vi "View Direction Write.vi"(6 "Control Ref Queue":T1, 8 "error in (no error)":errorcluster, 9 "View Direction":T2(ring), 11 "3D Plot.lvclass in":refnum<class "3D Plot.lvclass">) -> (0 "error out":errorcluster, 3 "3D Plot.lvclass out":refnum<class "3D Plot.lvclass">)   [LabVIEW 2020, in "3D Plot.lvclass"]
uses:
  3D Plot.lvclass
  3DMathPlot Ctrl Act Queue.ctl
  3DMathPlot Ctrl Act Cluster.ctl
  3DMathPlot State Class.ctl
  3D Plot.lvclass/3D Plot.ctl
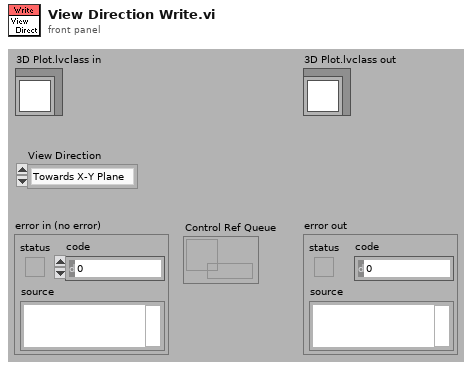
[diagram p1: front panel]
types:
  T1 = typedef "3DMathPlot Ctrl Act Queue.ctl" = refnum<queue>
  T2 = enum32{"Towards X-Y Plane", "Towards X-Z Plane", "Towards Y-Z Plane", "User Defined"}
  T3 = typedef "3DMathPlot Ctrl Act Cluster.ctl" = cluster{"3D Picture Control":refnum<vi>, "Render Window Refnum":refnum<vi>, "XY Graph":refnum<vi>, "Intensity Graph":refnum<vi>, "Color Legend Palette":refnum<vi>, "Projection Palette":refnum<vi>, "XControl  Ref":refnum<vi>, "Facade Ref":refnum<vi>, "Export Image Ref":refnum<vi>, "Clear Data Flag":bool, "Display State Change Class":T4}
  T4 = typedef "3DMathPlot State Class.ctl" = enum16{"Update All Objects (Undo)", "Update Light Object Only", "Update Axis Object Only", "Update Plot Object Only", "Update Cursor Object Only", "Update Axis Plot Cursor Objects", "No Update"}
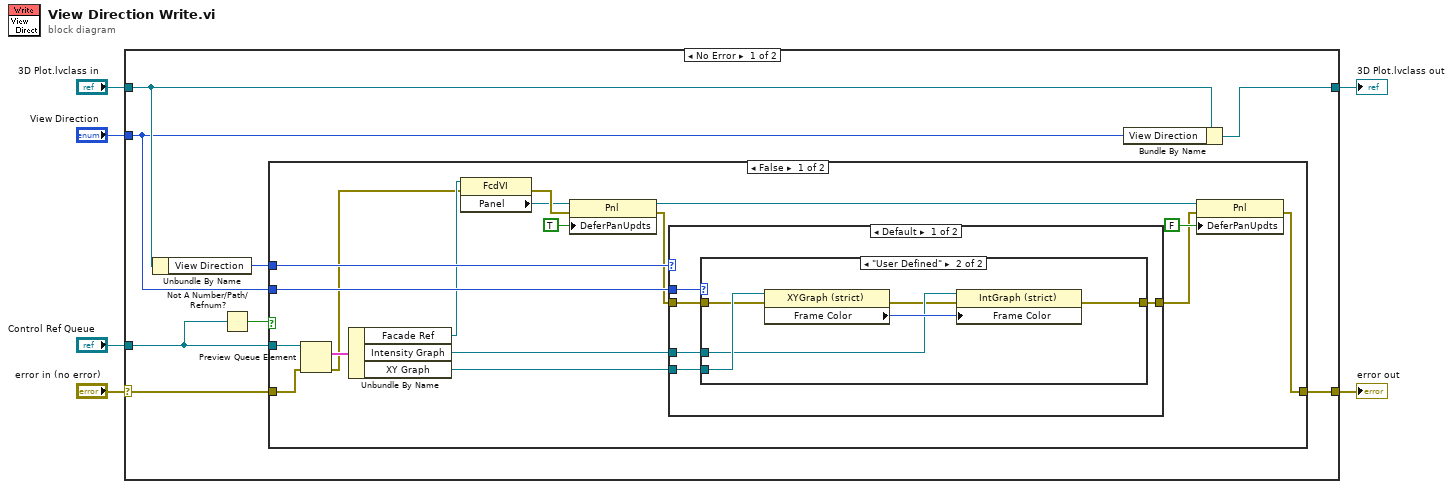
[diagram p0: block diagram]
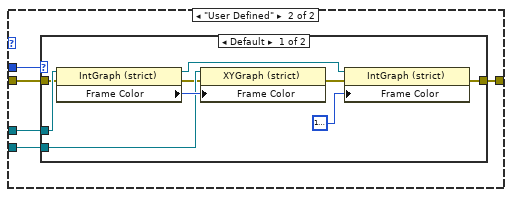
[diagram p3: hidden frame]
diagram:
  n1 = case shown="No Error" "error in (no error)" {
    selector: "error in (no error)" -> [w11 w60]
    tunnel: "View Direction" -> [w9 _]
    tunnel: "3D Plot.lvclass in" -> [w13 w61]
    tunnel: [w14 w61] -> w4
    tunnel: [w7 w60] -> w2
    tunnel: "Control Ref Queue" -> [w8 _]
    frame No Error {
      n2 = Unbundle By Name(w13) -> ("View Direction"=w10:T2)
      n3 = Not A Number/Path/Refnum?(number/path/refnum=w8) -> (NaN/Path/Refnum?=w12:bool)
      n4 = case shown="False" w12 {
        tunnel: w8 -> [w30 _]
        tunnel: w11 -> [w29 w59]
        tunnel: w10 -> [w28 _]
        tunnel: w9 -> [w27 _]
        tunnel: [w15 w59] -> w7
        frame False {
          n5 = Preview Queue Element(queue=w30, error in (no error)=w29) -> (element=w31:T3, error out=w18:errorcluster)  [unwired: 3 out]
          n6 = Unbundle By Name(w31) -> ("Facade Ref"=w23:refnum<vi>, "Intensity Graph"=w20:refnum<vi>, "XY Graph"=w19:refnum<vi>)
          n7 = property class="FcdVI"(reference=w23, error in=w18) -> (error out=w26:errorcluster, "Panel"=w24:refnum<vi>)  [unwired: 1 out]
          n8 = property class="Pnl"(reference=w24, error in=w26, "DeferPanUpdts"=TRUE ("Defer Panel Updates")) -> (reference out=w21:refnum<vi>, error out=w17:errorcluster)
          n9 = case shown="Default" w28 {
            tunnel: w27 -> [w36 w48]
            tunnel: w20 -> [w34 w47]
            tunnel: w19 -> [w35 w46]
            tunnel: w17 -> [w33 w45]
            tunnel: [w32 w44] -> w16
            frame Default {
              n10 = case shown="\"User Defined\"" w36 {
                tunnel: w35 -> [_ w42]
                tunnel: w34 -> [_ w41]
                tunnel: w33 -> [w37 w40]
                tunnel: [w37 w38] -> w32
                frame Default {
                }
                frame "User Defined" {
                  n11 = property class="XYGraph (strict)"(reference=w42, error in=w40) -> (error out=w39:errorcluster, "Frame Color"=w43:u32)  [unwired: 1 out]
                  n12 = property class="IntGraph (strict)"(reference=w41, error in=w39, "Frame Color"=w43) -> (error out=w38:errorcluster)  [unwired: 1 out]
                }
              }
            }
            frame "User Defined" {
              n13 = case shown="Default" w48 {
                tunnel: w47 -> [w57 _]
                tunnel: w46 -> [w55 _]
                tunnel: w45 -> [w54 w58]
                tunnel: [w49 w58] -> w44
                frame Default {
                  n14 = property class="IntGraph (strict)"(reference=w57, error in=w54) -> (reference out=w51:refnum<vi>, error out=w53:errorcluster, "Frame Color"=w56:u32)
                  n15 = property class="XYGraph (strict)"(reference=w55, error in=w53, "Frame Color"=w56) -> (error out=w50:errorcluster)  [unwired: 1 out]
                  n16 = property class="IntGraph (strict)"(reference=w51, error in=w50, "Frame Color"=u32 16777216) -> (error out=w49:errorcluster)  [unwired: 1 out]
                }
                frame "User Defined" {
                }
              }
            }
          }
          n17 = property class="Pnl"(reference=w21, error in=w16, "DeferPanUpdts"=FALSE ("Defer Panel Updates")) -> (error out=w15:errorcluster)  [unwired: 1 out]
        }
        frame True {
        }
      }
      n18 = Bundle By Name(cluster=w13, "View Direction"=w9) -> (w14:refnum<class "3D Plot.lvclass">)
    }
    frame Error {
    }
  }
  "3D Plot.lvclass out" <- w4
  "error out" <- w2
